vi "observacao.vi"() -> ()   [LabVIEW 2018, in "Shared_160.lvlib"] (continued)
                        n701 = call "Monta Comando.vi"("Comando"="ABRIR", "Dispositivo"="TRAPEIRA" ("Comando"), "Controlador"=w615) -> ()  [unwired: 2 in, 5 out]
                      }
                      frame True {
                        # "CLP Busy"
                        n702 = local read "TimeoutCUP"() -> (w618:u32)
                        n703 = call "TickTimeout.vi"("msInicial"=w618, "msTimeout"=u32 5000) -> ("Timeout"=w617:bool)  [unwired: 2 out]
                        n704 = case shown="True" w617 {
                          tunnel: [6 3] -> w616
                          frame False {
                          }
                          frame True {
                          }
                        }
                      }
                    }
                  }
                }
              }
              frame 7 {
                w622 = u16 15 items=["Alarme", "Atencao", "Erro", "Ocupado", "Plataforma", "LCB", "Trapeira", "Paravento", "DomoRap", "DomoCW", "DomoCCW", "TBD", "Em movimento", "TrapRUN", "TrapFCH", "TrapABT"] ("NomeStatus")
                # "Aqui também caberia um Timeout?"
                # "Aguarda abertura Trapeira"
                n705 = call "Bit Status CUP.vi"("NomeStatus"=w622) -> ("StatBit"=w623:bool)
                n706 = case shown="True" w623 {
                  tunnel: [7 0] -> w624
                  frame False {
                    # "Ainda movendo...\nAGUARDAR"
                  }
                  frame True {
                    # "Trapeira aberta.\nFIM"
                    n707 = call "TickTimeout.vi"() -> ("msTick"=w626:u32)  [unwired: 2 in, 2 out]
                    n708 = local write "Dome on Target"(TRUE ("Dome on Target")) -> ()
                    n709 = local write "TimeoutCUP"(w626) -> ()
                    n710 = global write "Global_Telescopio.vi" "T cup"(w626) -> ()
                  }
                }
              }
            }
            n711 = Equal To 0?(x=w493) -> (x = 0?=w492:bool)
            n712 = And(x=w492, y=w477) -> (x .and. y?=w488:bool)
            n713 = case shown="True" w488 {
              tunnel: w477 -> [w506 _]
              tunnel: [w505 "POINT" ("Boolean Text.Text")] -> w476
              frame False {
                n714 = case shown="True" w506 {
                  tunnel: ["POINT" ("Boolean Text.Text") "STOP" ("Boolean Text.Text")] -> w505
                  frame False {
                  }
                  frame True {
                  }
                }
              }
              frame True {
                w509 = TRUE
                # "MUDANÇA:\n22/6/2011 \nHab. Guider"
                n715 = local read "ChkDomeEnable"() -> (w510:bool)
                n716 = global write "Global_Telescopio.vi" "Botão GO = STOP"(FALSE) -> ()
                n717 = local write "LED GUIDER"(w509) -> ()
                n718 = local write "GUIDER"(w509) -> ()
                n719 = local write "DOME"(w510) -> ()
              }
            }
            n720 = Tick Count (ms)() -> (millisecond timer value=w469:u32)
            n721 = Subtract(x=w469, y=w475) -> (x-y=w468:u32)
            n722 = Less?(x=w468, y=w470) -> (x < y?=w471:bool)
            n723 = case shown="True" w471 {
              tunnel: w470 -> [_ w504]
              frame False {
              }
              frame True {
                n724 = Wait Until Next ms Multiple(millisecond multiple=w504) -> ()  [unwired: 1 out]
              }
            }
            n725 = control-ref of="BtTargetPoint"() -> (w503:refnum<vi>)
            n726 = call "PROTECAO.vi"("Estado In"=w481) -> ("Estado Out"=w480:i32)  [unwired: 2 in]
            n727 = property class="Bool"(reference=w503, "Boolean Text.Text"=w476) -> ()  [unwired: 1 in, 2 out]
            n728 = local write "statCUP"(w480) -> ()
            "statCUP 2" <- "statCUP"
            "Erro Lim" <- 15 ("y")
            "Erro PROTEC" <- 10 ("y")
          }
          frame #4 {
            # "CHECA FINAL DO APONTAMENTO"
            # "ascensão reta = tempo sideral - ângulo horário (2)"
            n729 = local read "LedPointing"() -> (w937:bool)
            n730 = case shown="True" w937 {
              frame False {
                n731 = property on="DOME" class="Bool (strict)"("Disabled"=u8 0) -> ()  [unwired: 2 in, 2 out]
              }
              frame True {
                n732 = local read "statCUP"() -> (w942:i32)
                n733 = local read "statAH"() -> (w941:i32)
                n734 = local read "statDEC"() -> (w943:i32)
                n735 = Compound Arithmetic op=ADD(w942, w941, w943) -> (w944:i32)
                n736 = Greater Than 0?(x=w944) -> (x > 0?=w940:bool)
                n737 = case shown="False" w940 {
                  selector: w940 -> [w945 _]
                  frame False {
                    w948 = TRUE
                    n738 = local read "ChkPointPrecessed"() -> (w946:bool)
                    n739 = local read "StrPointObjName"() -> (w951:string)
                    n740 = local read "StrPointObjRA"() -> (w950:string)
                    n741 = local read "StrPointObjDEC"() -> (w949:string)
                    n742 = local write "LedPointing"(w945) -> ()
                    n743 = property on="LedPointing" class="Bool (strict)"("Visible"=w945) -> ()  [unwired: 2 in, 2 out]
                    n744 = case shown="True" w946 {
                      tunnel: ["2000.000000000" ("Saída") w953] -> w947
                      frame False {
                        # "20240805"
                      }
                      frame True {
                        # "20240805"
                        n745 = call "Calcula epoch.vi"() -> ("epoch"=w956:dbl)  [unwired: 2 in]
                        n746 = Number To Fractional String(number=w956, precision (6)=i16 9) -> (F-format string=w954:string)  [unwired: 2 in]
                        n747 = call "Comma_to_Point.vi"("Lat_A"=w954) -> ("Saída"=w953:string)
                      }
                    }
                    n748 = global write "Global_Telescopio.vi" "NAME OBJETO"(w951) -> ()
                    n749 = global write "Global_Telescopio.vi" "DEC AQUIS"(w949) -> ()
                    n750 = global write "Global_Telescopio.vi" "RA AQUIS"(w950) -> ()
                    n751 = local write "Processa Centragem"(w948) -> ()
                    n752 = property on="LedPointWorkArea" class="Bool (strict)"("Visible"=w948) -> ()  [unwired: 2 in, 2 out]
                    n753 = global write "Global_Telescopio.vi" "EPOCH AQUIS"(w947) -> ()
                  }
                  frame True {
                  }
                }
              }
            }
            n754 = local read "VARIABLE \nTRACKING"() -> (w938:bool)
            n755 = case shown="True" w938 {
              frame False {
              }
              frame True {
                n756 = local write "DEC"("DECTARGET") -> ()
                n757 = local write "RA"("AHTARGET") -> ()
              }
            }
          }
          frame #5 {
            # "PROCESSO OBJETO CENTRADO"
            n758 = case shown="True" "Processa Centragem" {
              frame False {
              }
              frame True {
                w965 = u16 3 items=["Alarme", "Atencao", "Erro", "Ocupado", "Protecao", "Embreagem", "Tracking", "Var. Track", "Rápido", "Ligeiro", "Médio", "Lento", "Em movimento", ""] ("NomeStatus")
                w966 = u16 3 items=["Alarme", "Atencao", "Erro", "Ocupado", "Protecao", "Embreagem", "Tracking", "Var. Track", "Rápido", "Ligeiro", "Médio", "Lento", "Em movimento", ""] ("NomeStatus")
                # "Roda case interno quando \nos controladores AH e DEC\nestiverem desocupados."
                n759 = call "Bit Status AH.vi"("NomeStatus"=w966) -> ("StatBit"=w964:bool)
                n760 = call "Bit Status DEC.vi"("NomeStatus"=w965) -> ("StatBit"=w963:bool)
                n761 = Or(x=w964, y=w963) -> (x .or. y?=w960:bool)
                n762 = case shown="False" w960 {
                  selector: w960 -> [w985 _]
                  tunnel: "INDEXER" ("Comando") -> [w987 _]
                  tunnel: "ZERAR" ("Comando") -> [w986 _]
                  frame False {
                    w973 = u16 1 items=["ZERO", "AH", "DEC", "TUBO", "CUP"] ("Controlador")
                    w974 = u16 2 items=["ZERO", "AH", "DEC", "TUBO", "CUP"] ("Controlador")
                    w967 = 0.0 ("AcumAG DEC")
                    # "PROCESSOPRECESSÃO"
                    # "PROCESSO ZERA POS_MOTOR"
                    # "Precessão"
                    n763 = local read "PM_RA"() -> (w979:string)
                    n764 = local read "Temp amb"() -> (w982:string)
                    n765 = local read "hum local"() -> (w980:string)
                    n766 = local read "MeanDEC"() -> (w983:string)
                    n767 = local read "pressão atm"() -> (w981:string)
                    n768 = local read "MeanRA"() -> (w984:string)
                    n769 = local read "PM_DEC"() -> (w978:string)
                    n770 = call "Monta Comando.vi"("Comando"=w986, "Dispositivo"=w987, "Controlador"=w973) -> ()  [unwired: 2 in, 5 out]
                    n771 = call "Monta Comando.vi"("Comando"=w986, "Dispositivo"=w987, "Controlador"=w974) -> ()  [unwired: 2 in, 5 out]
                    n772 = call "PrecessFortran.vi"("Asc reta"=w984, "Var RA"=w979, "Declinação"=w983, "Temperatura (Kelvin)"=w982, "Pressao atmosferica (mB)"=w981, "Humidade relativa (0 a 1)"=w980, "Var DEC"=w978) -> ("Observed RA (radians)"=w977:dbl, "Observed Dec (radians)"=w976:dbl)  [unwired: 2 in, 5 out]
                    n773 = local write "Processa Centragem"(w985) -> ()
                    n774 = global write "Global_Telescopio.vi" "LatchPrecRA"(w977) -> ()
                    n775 = global write "Global_Telescopio.vi" "LatchPrecDEC"(w976) -> ()
                    n776 = global read "Global_Telescopio.vi" "Sideral Time"() -> (w970:dbl)
                    n777 = global read "Global_Telescopio.vi" "PosDEC"() -> (w972:dbl)
                    n778 = global read "Global_Telescopio.vi" "PosAH"() -> (w971:dbl)
                    n779 = Subtract(x=w970, y=w971) -> (x-y=w969:dbl)
                    n780 = local write "LatchDeslocDEC"(w972) -> ()
                    n781 = local write "LatchDeslocRA"(w969) -> ()
                    n782 = global write "Global_Telescopio.vi" "AcumPrecDEC"(w967) -> ()
                    n783 = global write "Global_Telescopio.vi" "LatchAG RA"(w967) -> ()
                    n784 = global write "Global_Telescopio.vi" "AcumAG DEC"(w967) -> ()
                    n785 = global write "Global_Telescopio.vi" "AcumPrecRA"(w967) -> ()
                    n786 = global write "Global_Telescopio.vi" "LatchAG DEC"(w967) -> ()
                    n787 = global write "Global_Telescopio.vi" "AcumAG RA"(w967) -> ()
                    n788 = global write "Global_Telescopio.vi" "ObjCentrado"(TRUE) -> ()
                    n789 = property on="Calagem" class="Bool"("Disabled"=u8 0) -> ()  [unwired: 2 in, 2 out]
                  }
                  frame True {
                  }
                }
              }
            }
          }
          frame #6 {
            w991 = u16 2 items=["Alarme", "Atencao", "Erro", "Ocupado", "TBD", "LCB", "Trapeira", "Paravento", "DomoRap", "DomoCW", "DomoCCW", "TBD", "Em movimento", "TBD"] ("NomeStatus")
            w992 = u16 3 items=["Alarme", "Atencao", "Erro", "Ocupado", "TBD", "LCB", "Trapeira", "Paravento", "DomoRap", "DomoCW", "DomoCCW", "TBD", "Em movimento", "TBD"] ("NomeStatus")
            w996 = u16 3 items=["Alarme", "Atencao", "Erro", "Ocupado", "Protecao", "Embreagem", "Tracking", "Var. Track", "Rápido", "Ligeiro", "Médio", "Lento", "Em movimento", ""] ("NomeStatus")
            w997 = u16 3 items=["Alarme", "Atencao", "Erro", "Ocupado", "Protecao", "Embreagem", "Tracking", "Var. Track", "Rápido", "Ligeiro", "Médio", "Lento", "Em movimento", ""] ("NomeStatus")
            w1005 = "ERROS" ("Comando")
            w1008 = u16 2 items=["Alarme", "Atencao", "Erro", "Ocupado", "Protecao", "Embreagem", "Tracking", "Var. Track", "Rápido", "Ligeiro", "Médio", "Lento", "Em movimento", ""] ("NomeStatus")
            w1009 = u16 2 items=["Alarme", "Atencao", "Erro", "Ocupado", "Protecao", "Embreagem", "Tracking", "Var. Track", "Rápido", "Ligeiro", "Médio", "Lento", "Em movimento", ""] ("NomeStatus")
            w1006 = "PROG" ("Comando")
            # "LOGTCS ERROS"
            n790 = call "Bit Status AH.vi"("NomeStatus"=w1009) -> ("StatBit"=w999:bool)
            n791 = call "Bit Status AH.vi"("NomeStatus"=w997) -> ("StatBit"=w995:bool)
            n792 = call "Bit Status DEC.vi"("NomeStatus"=w1008) -> ("StatBit"=w998:bool)
            n793 = call "Bit Status DEC.vi"("NomeStatus"=w996) -> ("StatBit"=w994:bool)
            n794 = call "Bit Status CUP.vi"("NomeStatus"=w991) -> ("StatBit"=w1007:bool)
            n795 = call "Bit Status CUP.vi"("NomeStatus"=w992) -> ("StatBit"=w1004:bool)
            n796 = Not(x=w1004) -> (.not. x?=w1003:bool)
            n797 = Not(x=w995) -> (.not. x?=w1001:bool)
            n798 = Not(x=w994) -> (.not. x?=w1002:bool)
            n799 = And(x=w1007, y=w1003) -> (x .and. y?=w990:bool)
            n800 = And(x=w999, y=w1001) -> (x .and. y?=w1000:bool)
            n801 = And(x=w998, y=w1002) -> (x .and. y?=w993:bool)
            n802 = And(x=FALSE, y=w990) -> (x .and. y?=w989:bool)
            n803 = case shown="True" w993 {
              selector: w993 -> [_ w1018]
              tunnel: w1006 -> [_ w1019]
              tunnel: w1005 -> [_ w1015]
              frame False {
              }
              frame True {
                w1016 = u16 2 items=["ZERO", "AH", "DEC", "TUBO", "CUP"] ("Controlador")
                n804 = call "Monta Comando.vi"("Comando"=w1015, "Dispositivo"=w1019, "Controlador"=w1016) -> ("Resposta"=w1017:string)  [unwired: 2 in, 4 out]
                n805 = call "Envia LOG.vi"("Error message"=w1017, "Controlador"=w1016, "Log de erro"=w1018) -> ()  [unwired: 5 in, 2 out]
              }
            }
            n806 = case shown="True" w989 {
              selector: w989 -> [_ w1013]
              tunnel: w1006 -> [_ w1014]
              tunnel: w1005 -> [_ w1010]
              frame False {
              }
              frame True {
                w1011 = u16 4 items=["ZERO", "AH", "DEC", "TUBO", "CUP"] ("Controlador")
                n807 = call "Monta Comando.vi"("Comando"=w1010, "Dispositivo"=w1014, "Controlador"=w1011) -> ("Resposta"=w1012:string)  [unwired: 2 in, 4 out]
                n808 = call "Envia LOG.vi"("Error message"=w1012, "Controlador"=w1011, "Log de erro"=w1013) -> ()  [unwired: 5 in, 2 out]
              }
            }
            n809 = case shown="True" w1000 {
              selector: w1000 -> [_ w1023]
              tunnel: w1006 -> [_ w1024]
              tunnel: w1005 -> [_ w1020]
              frame False {
              }
              frame True {
                w1021 = u16 1 items=["ZERO", "AH", "DEC", "TUBO", "CUP"] ("Controlador")
                n810 = call "Monta Comando.vi"("Comando"=w1020, "Dispositivo"=w1024, "Controlador"=w1021) -> ("Resposta"=w1022:string)  [unwired: 2 in, 4 out]
                n811 = call "Envia LOG.vi"("Error message"=w1022, "Controlador"=w1021, "Log de erro"=w1023) -> ()  [unwired: 5 in, 2 out]
              }
            }
          }
          frame #7 {
            # "MASSA DE AR"
            # "z'"
            # "z * (1 - 0,0012* (z* z -1) )"
            # "(z* z -1)"
            # "z"
            # "O Hour Angle é calculado com essa equação (AH = TS - RA), \nsendo TS o tempo sideral que você fica calculando o tempo todo e RA a \ncoordenada que vem do quadro TARGET da aba POINTING."
            # "Coslat"
            # "Sinlat"
            # "MASSA DE AR\n# define LAT -22,534444444444 / / Lat itude do telescópio\n# define SINLAT -0,383238771 / / Seno da Lat itude\n# define COSLAT 0,923649308 / / Cosseno da Lat itude\ndouble airmass (double ah, double delta) / / ângulos dos eixos AH e DEC em radianos\n{ double z;\nz = 1./ (SINLAT* sin(delta) + COSLAT* cos(delta) * cos(ah) ) ;\nz = z * (1 - 0,0012* (z* z -1) ) ;\nif (z > = 10) z = 9.999;\nif (z < 0) z = 0;\nreturn (z) ;\n}"
            n812 = global read "Global_Telescopio.vi" "AH_now"() -> (w1025:dbl)
            n813 = global read "Global_Telescopio.vi" "delta_now"() -> (w1026:dbl)
            n814 = Cosine(x=w1026) -> (cos(x)=w1046:dbl)
            n815 = Sine(x=w1026) -> (sin(x)=w1048:dbl)
            n816 = Cosine(x=w1025) -> (cos(x)=w1044:dbl)
            n817 = Multiply(x=0.923649308 ("Delta=DEC"), y=w1046) -> (x*y=w1045:dbl)
            n818 = Multiply(x=-0.383238771 ("Delta=DEC"), y=w1048) -> (x*y=w1043:dbl)
            n819 = Multiply(x=w1045, y=w1044) -> (x*y=w1042:dbl)
            n820 = Add(x=w1043, y=w1042) -> (x+y=w1041:dbl)
            n821 = Reciprocal(x=w1041) -> (1/x=w1033:dbl)
            n822 = Subtract(x=w1033, y=1.0) -> (x-y=w1039:dbl)
            n823 = Multiply(x=w1033, y=w1039) -> (x*y=w1038:dbl)
            n824 = Multiply(x=w1038, y=0.0012) -> (x*y=w1035:dbl)
            n825 = Subtract(x=1.0 ("y"), y=w1035) -> (x-y=w1034:dbl)
            n826 = Multiply(x=w1033, y=w1034) -> (x*y=w1030:dbl)
            n827 = Greater Or Equal?(x=w1030, y=10.0) -> (x >= y?=w1031:bool)
            n828 = case shown="True" w1031 {
              tunnel: [w1052 9.999999 ("y")] -> w1028
              tunnel: w1030 -> [w1052 _]
              frame False {
              }
              frame True {
              }
            }
            n829 = Less Than 0?(x=w1028) -> (x < 0?=w1029:bool)
            n830 = case shown="True" w1029 {
              tunnel: [w1050 0.0 ("y")] -> w1027
              tunnel: w1028 -> [w1050 _]
              frame False {
              }
              frame True {
              }
            }
            "Air Mass" <- w1027
            n831 = global write "Global_Telescopio.vi" "Air Mass"(w1027) -> ()
          }
          frame #8 {
          }
          frame #9 {
            # "20250707"
            # "ZeroMQ"
            # "ZeroMQ"
            # "CONDIÇÕES ATMOSFÉRICAS"
            # "A cada n Segundos\nEssa rotina gera 1\npulso!"
            # "Seg"
            # "Janela Das Condições Atmosféricas"
            n832 = property on="Weather data received" class="Bool (strict)"() -> ("Blinking"=w1056:bool)  [unwired: 2 in, 2 out]
            n833 = local write "Weather data received"(w1056) -> ()
            n834 = call "Get weather data.vi"() -> ("Wather160 data"=w1057:string[])  [unwired: 9 in]
            n835 = call "timepulse.vi"("de quantos segundos"=i16 10) -> ("PULSO"=w1061:bool)  [unwired: 2 in]
            n836 = call "Pulso_se_Mudou.vi"("Entrada"="Int/Ext") -> ("Saída"=w1059:bool)
            n837 = And(x="Int/Ext", y=w1061) -> (x .and. y?=w1058:bool)
            n838 = case shown="True" w1058 {
              tunnel: [TRUE TRUE ("Int/Ext")] -> w1055
              tunnel: w1059 -> [w1071 _]
              tunnel: w1057 -> [w1070 w1095]
              frame False {
                # "A chave Int/Ext mudou\npara pushbutton e é tratada apenas dentro deste case \"False\" nos períodos inativos de \"time pulse\" ligado ao terminal ? do case.\n\nOs valores internos (dew point, temperatura, umidade ) somente são mostrados enquanto a chave ficar pressionada pelo mouse.\n\nIsto garante o uso dos valores externos desssas grandezas no cálculo da precessão."
                n839 = case shown="True" w1071 {
                  tunnel: w1070 -> [_ w1072]
                  frame False {
                  }
                  frame True {
                    # "ZeroMQ"
                    # "Display"
                    # "ESTE CASO SOMENTE É EXECUTADO QUANDO A CHAVE INT/EXT MUDA DE ESTADO"
                    n840 = local read "Int/Ext"() -> (w1076:bool)
                    n841 = case shown="True" w1076 {
                      tunnel: [28 ("index") 5 ("index")] -> w1074
                      tunnel: [29 ("index") 6 ("index")] -> w1075
                      tunnel: [27 ("index") 2 ("index")] -> w1073
                      frame False {
                        # "Interno"
                      }
                      frame True {
                        # "Externo"
                      }
                    }
                    n842 = Index Array(array=w1072, index #1=w1073, index #2=w1074, index #3=w1075) -> (element #1=w1079:string, element #2=w1078:string, element #3=w1077:string)
                    n843 = call "point_to_comma.vi"("Lat_A"=w1079) -> ("Saída"=w1081:string)
                    n844 = call "point_to_comma.vi"("Lat_A"=w1078) -> ("Saída"=w1082:string)
                    n845 = call "point_to_comma.vi"("Lat_A"=w1077) -> ("Saída"=w1085:string)
                    n846 = Fract/Exp String To Number(string=w1081, default (0 dbl)=1.0 ("default (0 DBL)")) -> (number=w1086:dbl)  [unwired: 2 in, 1 out]
                    n847 = Fract/Exp String To Number(string=w1082, default (0 dbl)=1.0 ("default (0 DBL)")) -> (number=w1087:dbl)  [unwired: 2 in, 1 out]
                    n848 = Fract/Exp String To Number(string=w1085, default (0 dbl)=1.0 ("default (0 DBL)")) -> (number=w1088:dbl)  [unwired: 2 in, 1 out]
                    n849 = local write "Temperature"(w1086) -> ()
                    n850 = local write "Humidity"(w1087) -> ()
                    n851 = local write "Dew Point"(w1088) -> ()
                  }
                }
              }
              frame True {
                n852 = stacked-sequence {
                  tunnel: w1095 -> [_ w1115 _ _]
                  frame #0 {
                    # "O botão INT/ EXT (cf. figura 3) seleciona se os most radores TEMPERATURE, HUMIDITY\ne DEW POINT são atualizados com os valores internos ou externos desse regist ro.\nA barra gráfica CLOUSURE LIMITS deve ser deslocada em função da proximidade\n(dada por um valor percentural de zero a 100%) dos valores lidos do arquivo de dados\natmosféricos com os valores- limite das grandezas listadas nesse quadro. Para\nPRESSURE e WIND SPEED, considerar os valores- limite desse quadro como o final de\numa escala de 0 a 100%, cujo valor inicial (0%) corresponde ao valor zero dessas\ngrandezas. Para as grandezas DEWPOINT, interna e externa, considerar os valores\nlimites listados no quadro como final da escala (100%) e cada décimo de ºC acima\ndos valores- limite como 1% da escala."
                    # "A simulação da janela ENVIRONMENT STATUS será feita com os dados de um arquivo\ngerado pela estação meteorológica contendo os regist ros de 24 horas de monitoria,\nsendo cada regist ro efetuado em intervalos de 10 minutos. A simulação deve procurar\nnesse arquivo (anexo, LNA-TCSPD-MP-00012-01-100.txt ) o regist ro correspondente à\nhora local do PC, ler esse regist ro e ret irar as informações de cada most rador para\natualizar essa janela."
                  }
                  frame #1 {
                    w1139 = "\t"
                    # "ZeroMQ"
                    # "O Fortran usa valores\nde umidade entre 0 e 1."
                    # "MUDANÇA 08/04/2011:\nCriada a variável AtmosferaStr para guardar dados\nmeteorológicos para Erros de Apontamento"
                    # "Celsius -->Kelvin\nO Fortran usa Kelvin"
                    # "bar"
                    n853 = global read "Global_Telescopio.vi" "weather160 PUB time"() -> (→"Weather rec. time":timestamp)
                    n854 = case shown="True" TRUE {
                      tunnel: [27 ("index") 2 ("index")] -> w1133
                      tunnel: [28 ("index") 5 ("index")] -> w1132
                      tunnel: [29 ("index") 6 ("index")] -> w1131
                      frame False {
                        # "Interno"
                      }
                      frame True {
                        # "Externo"
                      }
                    }
                    n855 = global read "Global_Telescopio.vi" "Default Met"() -> (w1108:bool)
                    n856 = Index Array(array=w1115, index #1=w1133, index #2=w1132, index #3=w1131, index #4=7 ("index"), index #5=8 ("index"), index #6=12 ("index"), index #7=16 ("index"), index #8=2 ("index"), index #9=5 ("index"), index #10=27 ("index"), index #11=28 ("index"), index #12=35 ("index")) -> (element #1=w1164:string, element #2=w1176:string, element #3=w1173:string, element #4=w1169:string, element #5=w1140:string, element #6=w1168:string, element #7=w1113:string, element #8=w1112:string, element #9=w1111:string, element #10=w1150:string, element #11=w1149:string, element #12=w1134:string)
                    "Wind Dir" <- w1140
                    n857 = property on="Default" class="Str"("Visible"=w1108) -> ()  [unwired: 2 in, 2 out]
                    n858 = call "Weather data mabager.vi"("umidade in"=w1111, "temperatura in"=w1112, "pressao in"=w1113, "Default Met"=w1108) -> ("umidade out"=w1109:string, "temperatura out"=w1110:string, "pressao out"=w1114:string, "led on"=→"Weather data received":bool, "wather160 led state"=w1104:cluster{u32, u32}[], "blink"=w1105:bool)  [unwired: 2 out]
                    n859 = property on="Weather data received" class="Bool (strict)"("Colors [4]"=w1104) -> ()  [unwired: 2 in, 2 out]
                    n860 = property on="Weather data received" class="Bool (strict)"("Blinking"=w1105) -> ()  [unwired: 2 in, 2 out]
                    n861 = Decimal String To Number(string=w1134) -> (number=→"LEAF":i32)  [unwired: 2 in, 1 out]
                    n862 = call "point_to_comma.vi"("Lat_A"=w1164) -> ("Saída"=w1161:string)
                    n863 = call "point_to_comma.vi"("Lat_A"=w1176) -> ("Saída"=w1162:string)
                    n864 = call "point_to_comma.vi"("Lat_A"=w1173) -> ("Saída"=w1143:string)
                    n865 = call "point_to_comma.vi"("Lat_A"=w1169) -> ("Saída"=w1141:string)
                    n866 = call "point_to_comma.vi"("Lat_A"=w1168) -> ("Saída"=w1142:string)
                    n867 = call "point_to_comma.vi"("Lat_A"=w1114) -> ("Saída"=w1146:string)
                    "pressão atm" <- w1146
                    n868 = call "point_to_comma.vi"("Lat_A"=w1113) -> ("Saída"=w1117:string)
                    n869 = call "point_to_comma.vi"("Lat_A"=w1110) -> ("Saída"=w1148:string)
                    n870 = call "point_to_comma.vi"("Lat_A"=w1109) -> ("Saída"=w1147:string)
                    n871 = call "point_to_comma.vi"("Lat_A"=w1150) -> ("Saída"=w1145:string)
                    n872 = call "point_to_comma.vi"("Lat_A"=w1149) -> ("Saída"=w1144:string)
                    n873 = Concatenate Strings(w1148, w1139, w1147, w1139, w1146, w1139, w1145, w1139, w1144, w1139, w1143, w1139, w1141, w1139, w1140, w1139) -> (→"AtmosferaStr":string)
                    n874 = Fract/Exp String To Number(string=w1117, default (0 dbl)=1.0 ("default (0 DBL)")) -> (number=→"Pressure":dbl)  [unwired: 2 in, 1 out]
                    n875 = Fract/Exp String To Number(string=w1161, default (0 dbl)=1.0 ("default (0 DBL)")) -> (number=→"Temperature":dbl)  [unwired: 2 in, 1 out]
                    n876 = Fract/Exp String To Number(string=w1162, default (0 dbl)=1.0 ("default (0 DBL)")) -> (number=→"Humidity":dbl)  [unwired: 2 in, 1 out]
                    n877 = Fract/Exp String To Number(string=w1143, default (0 dbl)=1.0 ("default (0 DBL)")) -> (number=→"Dew Point":dbl)  [unwired: 2 in, 1 out]
                    n878 = Fract/Exp String To Number(string=w1141, default (0 dbl)=1.0 ("default (0 DBL)")) -> (number=→"Wind Speed":dbl)  [unwired: 2 in, 1 out]
                    n879 = Fract/Exp String To Number(string=w1142, default (0 dbl)=1.0 ("default (0 DBL)")) -> (number=→"Wind Chill":dbl)  [unwired: 2 in, 1 out]
                    n880 = Fract/Exp String To Number(string=w1146, default (0 dbl)=1.0 ("default (0 DBL)")) -> (number=w1135:dbl)  [unwired: 2 in, 1 out]
                    n881 = Fract/Exp String To Number(string=w1148, default (0 dbl)=1.0 ("default (0 DBL)")) -> (number=w1120:dbl)  [unwired: 2 in, 1 out]
                    n882 = Fract/Exp String To Number(string=w1147, default (0 dbl)=1.0 ("default (0 DBL)")) -> (number=w1119:dbl)  [unwired: 2 in, 1 out]
                    n883 = Add(x=w1120, y=273.5 ("default (0 DBL)")) -> (x+y=w1159:dbl)
                    n884 = Divide(x=w1119, y=100.0 ("default (0 DBL)")) -> (x/y=w1153:dbl)
                    n885 = global write "Global_Telescopio.vi" "BAR"(w1135) -> ()
                    n886 = global write "Global_Telescopio.vi" "HUM"(w1119) -> ()
                    n887 = global write "Global_Telescopio.vi" "TEMP"(w1120) -> ()
                    n888 = Number To Fractional String(number=w1159, precision (6)=i16 1) -> (F-format string=→"Temp amb":string)  [unwired: 2 in]
                    n889 = Number To Fractional String(number=w1153, precision (6)=i16 2) -> (F-format string=→"hum local":string)  [unwired: 2 in]
                    n890 = call "Alarme_Atmosferico.vi"("Internal Dew Point"="Internal Dew Point", "Dew Point"="Dew Point 2", "Humidity"="Humidity 2", "Wind Speed"="Wind Speed 2", "LEAF"="LEAF 2") -> ("PUB alarme atmosferico"=w1097:string)  [unwired: 6 in]
                    n891 = global write "Global_Telescopio.vi" "PUB AtmAlarme"(w1097) -> ()
                  }
                  frame #2 {
                    # "Em relação as suas perguntas:\n- Temperaturas (Temperature, Dew Point e Wind Chill): mínimo/máximo: -20 a +50 graus\n- Humidity:  0 a 100%\n- Pressão atmosférica: de 300 a 1200 mBar\n- Velocidade do vento: 0 a 300 Km/h\n\nNotar que a chave INT/EXT na parte superior do quadro \nesquerdo seleciona se são mostrados os valores internos ou externos de Temperatura, Umidade e Dew Point."
                    # "Pressure Max"
                    # "Wind chill Point Max"
                    # "Temp Point Max"
                    # "Dew Point Max"
                    # "Humidity Max"
                    # "Speed Max"
                    # "Steady Wind           >  70 Km/h\nRelative Humidity    >  97 %\nInternal Dewpoint  <  0.5  C\nExternal Dewpoint <  1.0  C"
                    n892 = Divide(x=100.0, y=300.0 ("x")) -> (x/y=w1214:dbl)
                    n893 = Divide(x=100.0, y=100.0 ("x")) -> (x/y=w1208:dbl)
                    n894 = Divide(x=100.0, y=50.0 ("x")) -> (x/y=w1206:dbl)
                    n895 = Divide(x=100.0, y=50.0 ("x")) -> (x/y=w1200:dbl)
                    n896 = Divide(x=100.0, y=50.0 ("x")) -> (x/y=w1199:dbl)
                    n897 = Divide(x=100.0, y=1200.0 ("x")) -> (x/y=w1194:dbl)
                    n898 = local read "Temperature"() -> (w1191:dbl)
                    n899 = local read "Wind Speed"() -> (w1213:dbl)
                    n900 = local read "Wind Chill"() -> (w1192:dbl)
                    n901 = local read "Dew Point"() -> (w1203:dbl)
                    n902 = local read "Humidity"() -> (w1207:dbl)
                    n903 = local read "Pressure"() -> (w1193:dbl)
                    n904 = Multiply(x=w1213, y=w1214) -> (x*y=w1190:dbl)
                    n905 = Multiply(x=w1207, y=w1208) -> (x*y=w1189:dbl)
                    n906 = Multiply(x=w1203, y=w1206) -> (x*y=w1188:dbl)
                    n907 = Multiply(x=w1191, y=w1200) -> (x*y=w1187:dbl)
                    n908 = Multiply(x=w1192, y=w1199) -> (x*y=w1186:dbl)
                    n909 = Multiply(x=w1193, y=w1194) -> (x*y=w1185:dbl)
                    n910 = Build Array(w1190, w1189, w1188, w1187, w1186, w1185) -> (w1184:dbl[])
                    n911 = Array Max & Min(array=w1184) -> (max value=w1183:dbl)  [unwired: 3 out]
                    n912 = local write "SlideEnviromental"(w1183) -> ()
                  }
                  frame #3 {
                    # "Determinadas as proximidades de cada grandeza em valores percentuais, selecionar o\nvalor da mais elevada para ser most rado na barra gráfica. A cor dessa barra gráfica\ndeve mudar em função do valor most rado. Enquanto est iver abaixo de 90%, ela deve\nser verde, ent re 90 e 95% amarela e acima de 95% vermelha. O led ao lado desse\nbarra deve ficar ligado e ter a mesma cor da barra gráfica, mas quando esta\nult rapassar 90%, ou seja quando for amarela ou vermelha, o led deve piscar."
                    n913 = local read "SlideEnviromental"() -> (w1215:dbl)
                    n914 = In Range and Coerce(upper limit=95.0 ("lower limit"), x=w1215, lower limit=90.0 ("upper limit")) -> (In Range?=w1220:bool)  [unwired: 1 out]
                    n915 = Less?(x=w1215, y=90.0) -> (x < y?=w1222:bool)
                    n916 = Greater?(x=w1215, y=95.0 ("lower limit")) -> (0:w1219:bool)
                    n917 = case shown="True" w1220 {
                      frame False {
                      }
                      frame True {
                        n918 = stacked-sequence {
                          frame #0 {
                            n919 = property on="SlideEnviromental" class="Slide (strict)"("Fill Color"=u32 16772882) -> ()  [unwired: 2 in, 2 out]
                            n920 = local write "Boolean 11"(TRUE ("Boolean 11")) -> ()
                            n921 = property on="Boolean 11" class="Bool (strict)"("Blinking"=FALSE) -> ()  [unwired: 2 in, 2 out]
                          }
                          frame #1 {
                            # "Cor do Led"
                            # "lig"
                            # "des"
                            n922 = Bundle(u32 7171459, u32 46096) -> (w1242:cluster{u32, u32})  [unwired: 1 in]
                            n923 = Bundle(u32 16772882, u32 46096) -> (w1241:cluster{u32, u32})  [unwired: 1 in]
                            n924 = Build Array(w1242, w1241) -> (w1240:cluster{u32, u32}[])
                            n925 = property on="Boolean 11" class="Bool (strict)"("Colors [4]"=w1240) -> ()  [unwired: 2 in, 2 out]
                          }
                        }
                      }
                    }
                    n926 = case shown="True" w1222 {
                      frame False {
                      }
                      frame True {
                        n927 = stacked-sequence {
                          frame #0 {
                            n928 = property on="SlideEnviromental" class="Slide (strict)"("Fill Color"=u32 6618880) -> ()  [unwired: 2 in, 2 out]
                            n929 = local write "Boolean 11"(TRUE ("Boolean 11")) -> ()
                            n930 = property on="Boolean 11" class="Bool (strict)"("Blinking"=FALSE) -> ()  [unwired: 2 in, 2 out]
                          }
                          frame #1 {
                            # "Cor do Led"
                            # "lig"
                            # "des"
                            n931 = Bundle(u32 7171459, u32 46096) -> (w1246:cluster{u32, u32})  [unwired: 1 in]
                            n932 = Bundle(u32 6618880, u32 46096) -> (w1247:cluster{u32, u32})  [unwired: 1 in]
                            n933 = Build Array(w1246, w1247) -> (w1248:cluster{u32, u32}[])
                            n934 = property on="Boolean 11" class="Bool (strict)"("Colors [4]"=w1248) -> ()  [unwired: 2 in, 2 out]
                          }
                        }
                      }
                    }
                    n935 = case shown="True" w1219 {
                      frame False {
                      }
                      frame True {
                        n936 = stacked-sequence {
                          frame #0 {
                            n937 = local write "Boolean 11"(TRUE ("Boolean 11")) -> ()
                            n938 = property on="SlideEnviromental" class="Slide (strict)"("Fill Color"=u32 16715776) -> ()  [unwired: 2 in, 2 out]
                            n939 = property on="Boolean 11" class="Bool (strict)"("Blinking"=TRUE) -> ()  [unwired: 2 in, 2 out]
                          }
                          frame #1 {
                            # "Cor do Led"
                            # "lig"
                            # "des"
                            n940 = Bundle(u32 7171459, u32 46096) -> (w1226:cluster{u32, u32})  [unwired: 1 in]
                            n941 = Bundle(u32 16715776, u32 46096) -> (w1227:cluster{u32, u32})  [unwired: 1 in]
                            n942 = Build Array(w1226, w1227) -> (w1228:cluster{u32, u32}[])
                            n943 = property on="Boolean 11" class="Bool (strict)"("Colors [4]"=w1228) -> ()  [unwired: 2 in, 2 out]
                          }
                        }
                      }
                    }
                  }
                }
              }
            }
            n944 = global read "Global_Telescopio.vi" "BtShutCloseSimul"() -> (w1054:bool)
            n945 = case shown="True" w1054 {
              frame False {
              }
              frame True {
                # "Escreve no LOG o estado do shutter"
                n946 = global write "Global_Telescopio.vi" "BtShutCloseSimul"(FALSE) -> ()
                n947 = call "Log_Shutter.vi"("command"=" ", "domeState"="CLOSED " ("command"), "pathLogDomeFile"="C:\\TCS\\LOG\\SHUTTER\\SHUTTER.TXT" ("pathLogFocoString")) -> ()  [unwired: 6 in]
              }
            }
            n948 = flat-sequence {
              tunnel: w1055 -> [_]
              frame #0 {
                n949 = local read "LEAF"() -> (w1068:i32)
                n950 = call "Testa_Leaf.vi"("enable"=TRUE, "LEAF"=w1068) -> ()  [unwired: 10 in]
              }
            }
          }
          frame #10 {
            w1276 = u16 3 items=["Alarme", "Atencao", "Erro", "Ocupado", "Protecao", "Embreagem", "Tracking", "Var. Track", "Rápido", "Ligeiro", "Médio", "Lento", "Em movimento", ""] ("NomeStatus")
            w1277 = u16 3 items=["Alarme", "Atencao", "Erro", "Ocupado", "Protecao", "Embreagem", "Tracking", "Var. Track", "Rápido", "Ligeiro", "Médio", "Lento", "Em movimento", ""] ("NomeStatus")
            # "20250728"
            # "PROCESSO AUTO GUIDER E NON-SIDERAL TRACKING"
            n951 = local read "ExternalTracking"() -> (w1259:bool)
            n952 = local read "VARIABLE \nTRACKING"() -> (w1254:bool)
            "LED VAR TRACKING" <- w1254
            n953 = global read "Global_Telescopio.vi" "ExtDEC correction"() -> (w1263:bool)
            n954 = global read "Global_Telescopio.vi" "ExtRA correction"() -> (w1262:bool)
            n955 = local read "MOUNT"() -> (w1269:bool)
            n956 = global read "Global_Telescopio.vi" "Correção Guider"() -> (w1273:bool)
            n957 = local read "LedPointing"() -> (w1275:bool)
            n958 = local read "MOVING"() -> (w1274:bool)
            n959 = call "Bit Status AH.vi"("NomeStatus"=w1277) -> ("StatBit"=w1266:bool)
            n960 = call "Bit Status DEC.vi"("NomeStatus"=w1276) -> ("StatBit"=w1265:bool)
            n961 = Not Or(1:w1265, 2:w1266) -> (0:w1270:bool)
            n962 = Not(x=w1274) -> (.not. x?=w1267:bool)
            n963 = Not(x=w1275) -> (.not. x?=w1268:bool)
            n964 = And(x=w1259, y=w1254) -> (x .and. y?=w1253:bool)
            "externalNST" <- w1253
            n965 = Or(x=w1263, y=w1262) -> (x .or. y?=w1264:bool)
            n966 = Not(x=w1259) -> (.not. x?=w1271:bool)
            n967 = global write "Global_Telescopio.vi" "PUB activeNST"(w1253) -> ()
            n968 = Compound Arithmetic op=AND(w1273, w1268, w1267, "GUIDER", w1269, w1270, w1271) -> (w1261:bool)
            n969 = Compound Arithmetic op=AND(w1269, w1268, w1267, w1259, w1254, w1264) -> (w1260:bool)
            n970 = case shown="True" w1261 {
              tunnel: w1260 -> [w1284 _]
              tunnel: w1266 -> [w1283 _]
              tunnel: w1265 -> [w1282 _]
              tunnel: w1263 -> [w1281 _]
              tunnel: w1262 -> [w1280 _]
              frame False {
                # "Reseta Flag da comunicação do Guider"
                # "CKECK FOR NON-SIDERAL TRACKING CORRECTIONS"
                n971 = case shown="True" w1284 {
                  tunnel: w1283 -> [_ w1291]
                  tunnel: w1282 -> [_ w1290]
                  tunnel: w1281 -> [_ w1289]
                  tunnel: w1280 -> [_ w1288]
                  frame False {
                    # "AO CONTRÁRIO DA CORREÇÃO GUIDER, O FLAG EXTERNAL CORRECTION NÃO DEVE SER APAGADO\nPARA SE TENTAR EXECUTAR A CORREÇÃO MAIS TARDE,, PARA NÃO PERDER O DESLOCAMENTO."
                    # "EXTERNAL NON-SIDERAL TRACKING DISABLED OR TELESCOPE NOT READY"
                  }
                  frame True {
                    # "EXTERNAL NON-SIDERAL TRACKING"
                    n972 = Not(x=w1291) -> (.not. x?=w1287:bool)
                    n973 = Not(x=w1290) -> (.not. x?=w1286:bool)
                    n974 = stacked-sequence {
                      tunnel: w1287 -> [w1294 _]
                      tunnel: w1286 -> [_ w1308]
                      tunnel: w1289 -> [_ w1309]
                      tunnel: w1288 -> [w1293 _]
                      frame #0 {
                        n975 = And(x=w1294, y=w1293) -> (x .and. y?=w1292:bool)
                        n976 = case shown="True" w1292 {
                          frame False {
                          }
                          frame True {
                            w1303 = u16 1 items=["ZERO", "AH", "DEC", "TUBO", "CUP"] ("Controlador")
                            # "MOVE TELESCÓPIO"
                            n977 = global read "Global_Telescopio.vi" "ExtRA_shift"() -> (w1299:string)
                            n978 = property on="Calagem" class="Bool"("Disabled"=u8 2) -> ()  [unwired: 2 in, 2 out]
                            n979 = call "Monta Comando.vi"("Set Point"=w1299, "Comando"="SHIFT", "Dispositivo"="EIXO" ("Comando"), "Controlador"=w1303) -> ("Erro Resp"=w1296:bool)  [unwired: 1 in, 4 out]
                            n980 = call "point_to_comma.vi"("Lat_A"=w1299) -> ("Saída"=w1298:string)
                            n981 = local read "Offset RA"() -> (w1301:dbl)
                            n982 = Fract/Exp String To Number(string=w1298) -> (number=w1297:dbl)  [unwired: 3 in, 1 out]
                            n983 = Add(x=w1297, y=w1301) -> (x+y=w1295:dbl)
                            n984 = case shown="False" w1296 {
                              selector: w1296 -> [w1305 _]
                              tunnel: w1295 -> [w1306 _]
                              frame False {
                                # "RESPOSTA ACK"
                                n985 = global write "Global_Telescopio.vi" "ExtRA correction"(w1305) -> ()
                                n986 = local write "Offset RA"(w1306) -> ()
                              }
                              frame True {
                                # "NAK"
                              }
                            }
                          }
                        }
                      }
                      frame #1 {
                        n987 = And(x=w1308, y=w1309) -> (x .and. y?=w1307:bool)
                        n988 = case shown="True" w1307 {
                          frame False {
                          }
                          frame True {
                            w1318 = u16 2 items=["ZERO", "AH", "DEC", "TUBO", "CUP"] ("Controlador")
                            # "MOVE TELESCÓPIO"
                            n989 = global read "Global_Telescopio.vi" "ExtDEC_shift"() -> (w1313:string)
                            n990 = property on="Calagem" class="Bool"("Disabled"=u8 2) -> ()  [unwired: 2 in, 2 out]
                            n991 = local read "Offset DEC"() -> (w1316:dbl)
                            n992 = call "Monta Comando.vi"("Set Point"=w1313, "Comando"="SHIFT", "Dispositivo"="EIXO" ("Comando"), "Controlador"=w1318) -> ("Erro Resp"=w1311:bool)  [unwired: 1 in, 4 out]
                            n993 = call "point_to_comma.vi"("Lat_A"=w1313) -> ("Saída"=w1314:string)
                            n994 = Fract/Exp String To Number(string=w1314) -> (number=w1312:dbl)  [unwired: 3 in, 1 out]
                            n995 = Add(x=w1312, y=w1316) -> (x+y=w1310:dbl)
                            n996 = case shown="False" w1311 {
                              selector: w1311 -> [w1320 _]
                              tunnel: w1310 -> [w1321 _]
                              frame False {
                                # "RESPOSTA ACK"
                                n997 = global write "Global_Telescopio.vi" "ExtDEC correction"(w1320) -> ()
                                n998 = local write "Offset DEC"(w1321) -> ()
                              }
                              frame True {
                                # "NAK"
                              }
                            }
                          }
                        }
                      }
                    }
                  }
                }
                n999 = global write "Global_Telescopio.vi" "Correção Guider"(FALSE ("Correção Guider")) -> ()
              }
              frame True {
                # "MUDANÇA:\n(25/08/2010)"
                # "É necessário testar se as\nstrings são igual a espaço\nem virtude de um BUG,\nno Soft do Auto guider!"
                # "TRADITIONAL GUIDING USING AUTOGUIDER"
                n1000 = global read "Global_Telescopio.vi" "guide_dir_ns"() -> (w1327:string)
                n1001 = global read "Global_Telescopio.vi" "guide_dir_we"() -> (w1328:string)
                n1002 = case shown="\"W\"" w1328 {
                  tunnel: [0.0 ("PreciseOffsetDEC 2") 1.0 ("PreciseOffsetDEC 2") -1.0 ("PreciseOffsetDEC 2")] -> w1325
                  frame " ", Default {
                  }
                  frame "W" {
                  }
                  frame "E" {
                  }
                }
                n1003 = case shown="\"N\"" w1327 {
                  tunnel: [0.0 ("PreciseOffsetDEC 2") 1.0 ("PreciseOffsetDEC 2") -1.0 ("PreciseOffsetDEC 2")] -> w1324
                  frame " ", Default {
                  }
                  frame "N" {
                  }
                  frame "S" {
                  }
                }
                n1004 = Equal To 0?(x=w1324) -> (x = 0?=w1323:bool)
                n1005 = Equal To 0?(x=w1325) -> (x = 0?=w1322:bool)
                n1006 = And(x=w1322, y=w1323) -> (x .and. y?=w1326:bool)
                n1007 = case shown="True" w1326 {
                  tunnel: w1325 -> [w1333 _]
                  tunnel: w1324 -> [w1332 _]
                  frame False {
                    # "Comandos do Auto guider contendo direção"
                    n1008 = global read "Global_Telescopio.vi" "esc_placa"() -> (w1331:string)
                    n1009 = Fract/Exp String To Number(use system decimal point (T)=FALSE, string=w1331) -> (number=w1330:dbl)  [unwired: 2 in, 1 out]
                    n1010 = stacked-sequence {
                      tunnel: w1333 -> [w1339 _ _]
                      tunnel: w1332 -> [_ w1359 _]
                      tunnel: w1330 -> [w1336 w1356 _]
                      frame #0 {
                        n1011 = global read "Global_Telescopio.vi" "guide_asc"() -> (w1338:dbl)
                        n1012 = local read "AtualDEC"() -> (w1344:dbl)
                        n1013 = global read "Global_Telescopio.vi" "CorrecaoMin"() -> (w1334:dbl)
                        n1014 = Cosine(x=w1344) -> (cos(x)=w1343:dbl)
                        n1015 = Multiply(x=w1338, y=w1336) -> (x*y=w1337:dbl)
                        n1016 = Absolute Value(x=w1343) -> (abs(x)=w1342:dbl)
                        n1017 = Divide(x=w1337, y=w1342) -> (x/y=w1340:dbl)
                        n1018 = Multiply(x=w1339, y=w1340) -> (x*y=w1335:dbl)
                        n1019 = Greater?(x=w1340, y=w1334) -> (0:w1341:bool)
                        n1020 = case shown="True" w1341 {
                          tunnel: w1335 -> [_ w1346]
                          frame False {
                          }
                          frame True {
                            w1350 = u16 1 items=["ZERO", "AH", "DEC", "TUBO", "CUP"] ("Controlador")
                            # "PROCESSO MOVE TELESCÓPIO"
                            n1021 = local read "Offset RA"() -> (w1347:dbl)
                            n1022 = Add(x=w1346, y=w1347) -> (x+y=w1348:dbl)
                            n1023 = property on="Calagem" class="Bool"("Disabled"=u8 2) -> ()  [unwired: 2 in, 2 out]
                            n1024 = call "Conversao Ms to Hora texto.vi"("TRUE=HORA\nFALSE=GRAU"=TRUE ("TRUE=HORA\nFALSE=GRAU"), "PrecDEC"=w1346) -> ("Hora/Graus Texto Decimal"=w1353:string)
                            n1025 = local write "Offset RA"(w1348) -> ()
                            n1026 = call "Monta Comando.vi"("Set Point"=w1353, "Comando"="MOVER_REL", "Dispositivo"="EIXO" ("Comando"), "Controlador"=w1350) -> ()  [unwired: 1 in, 5 out]
                          }
                        }
                      }
                      frame #1 {
                        n1027 = global read "Global_Telescopio.vi" "guide_dec"() -> (w1358:dbl)
                        n1028 = Multiply(x=w1358, y=w1356) -> (x*y=w1357:dbl)
                        n1029 = global read "Global_Telescopio.vi" "CorrecaoMin"() -> (w1354:dbl)
                        n1030 = Greater?(x=w1357, y=w1354) -> (0:w1360:bool)
                        n1031 = Multiply(x=w1359, y=w1357) -> (x*y=w1355:dbl)
                        n1032 = case shown="True" w1360 {
                          tunnel: w1355 -> [_ w1362]
                          frame False {
                          }
                          frame True {
                            w1366 = u16 2 items=["ZERO", "AH", "DEC", "TUBO", "CUP"] ("Controlador")
                            # "PROCESSO MOVE TELESCÓPIO"
                            n1033 = local read "Offset DEC"() -> (w1363:dbl)
                            n1034 = Add(x=w1362, y=w1363) -> (x+y=w1364:dbl)
                            n1035 = property on="Calagem" class="Bool"("Disabled"=u8 2) -> ()  [unwired: 2 in, 2 out]
                            n1036 = call "Conversao Ms to Hora texto.vi"("TRUE=HORA\nFALSE=GRAU"=FALSE ("TRUE=HORA\nFALSE=GRAU"), "PrecDEC"=w1362) -> ("Hora/Graus Texto Decimal"=w1369:string)
                            n1037 = local write "Offset DEC"(w1364) -> ()
                            n1038 = call "Monta Comando.vi"("Set Point"=w1369, "Comando"="MOVER_REL", "Dispositivo"="EIXO" ("Comando"), "Controlador"=w1366) -> ()  [unwired: 1 in, 5 out]
                          }
                        }
                      }
                      frame #2 {
                        # "Reseta Flag da comunicação do Guider"
                        n1039 = global write "Global_Telescopio.vi" "Correção Guider"(FALSE ("Correção Guider")) -> ()
                      }
                    }
                  }
                  frame True {
                    # "20250728"
                    n1040 = global write "Global_Telescopio.vi" "Correção Guider"(FALSE ("Correção Guider")) -> ()
                  }
                }
              }
            }
            n1041 = call "Borda Subida.vi"("Entrada"=w1253) -> ("Boolean"=w1258:bool)  [unwired: 4 in]
            n1042 = Select(t=T5."Disabled and Grayed Out" ("Disabled"), s=w1254, f=T5."Enabled" ("Disabled")) -> (s? t:f=w1256:T5)
            n1043 = property on="ExternalTracking" class="Bool (strict)"("DisabledEnum"=w1256) -> ()  [unwired: 2 in, 2 out]
            n1044 = case shown="True" w1258 {
              frame False {
              }
              frame True {
                n1045 = local write "Offset RA"(0.0 ("Offset RA")) -> ()
                n1046 = local write "Offset DEC"(0.0 ("Offset DEC")) -> ()
              }
            }
            "LED GUIDER" <- "GUIDER"
          }
          frame #11 {
            w1387 = u16 12 items=["Alarme", "Atencao", "Erro", "Ocupado", "Protecao", "Embreagem", "Tracking", "Var. Track", "Rápido", "Ligeiro", "Médio", "Lento", "Em movimento", ""] ("NomeStatus")
            w1386 = u16 12 items=["Alarme", "Atencao", "Erro", "Ocupado", "Protecao", "Embreagem", "Tracking", "Var. Track", "Rápido", "Ligeiro", "Médio", "Lento", "Em movimento", ""] ("NomeStatus")
            # "Aqui era a Global\nLIMITE"
            # "Este teste deve ser executado antes do Frame de enviar\ncomando do sistema de aquisição, em virtude de teste do \nmovimento."
            # "Quando o Movimento Parar\nreseta a Variável/Flag para enviar \no CR ao sitema de Aquisição"
            n1047 = global read "Global_Telescopio.vi" "AQ Offset Mov"() -> (w1383:bool)
            n1048 = call "Bit Status AH.vi"("NomeStatus"=w1386) -> ("StatBit"=w1389:bool)
            n1049 = call "Bit Status DEC.vi"("NomeStatus"=w1387) -> ("StatBit"=w1388:bool)
            n1050 = local read "Proteção"() -> (w1379:bool)
            n1051 = Not Or(1:w1388, 2:w1389) -> (0:w1384:bool)
            n1052 = case shown="True" w1379 {
              selector: w1379 -> [w1390 w1391]
              frame False {
                n1053 = local write "LIMITE"(w1390) -> ()
                n1054 = property on="LIMITE" class="Bool"("Blinking"=w1390) -> ()  [unwired: 2 in, 2 out]
              }
              frame True {
                n1055 = property on="LIMITE" class="Bool"("Blinking"=w1391) -> ()  [unwired: 2 in, 2 out]
                "LIMITE" <- w1391
              }
            }
            n1056 = And(x=w1383, y=w1384) -> (x .and. y?=w1385:bool)
            n1057 = case shown="True" w1385 {
              frame False {
              }
              frame True {
                n1058 = global write "Global_Telescopio.vi" "AQ Offset Mov"(FALSE ("AQ Offset Mov")) -> ()
              }
            }
            n1059 = global read "Global_Telescopio.vi" "Z_SEGURANÇA_GRAUS"() -> (w1382:dbl)
            n1060 = global read "Global_Telescopio.vi" "Zenital angle GRAUS"() -> (w1381:dbl)
            n1061 = global read "Global_Telescopio.vi" "FinalsFileDownload"() -> (→"Precess Data out-of-date":bool)
            n1062 = Greater?(x=w1381, y=w1382) -> (0:→"Security Zone":bool)
          }
          frame #12 {
            w1406 = u16 8 items=["Alarme", "Atencao", "Erro", "Ocupado", "Protecao", "Embreagem", "Tracking", "Var. Track", "Rápido", "Ligeiro", "Médio", "Lento", "Em movimento", ""] ("NomeStatus")
            w1407 = u16 8 items=["Alarme", "Atencao", "Erro", "Ocupado", "Protecao", "Embreagem", "Tracking", "Var. Track", "Rápido", "Ligeiro", "Médio", "Lento", "Em movimento", ""] ("NomeStatus")
            # "TU safe"
            # "ATUALIZAÇÃO DO QUADRO STATUS INFORMATION"
            n1063 = call "Bit Status DEC.vi"("NomeStatus"=w1406) -> ("StatBit"=w1404:bool)
            n1064 = call "Bit Status AH.vi"("NomeStatus"=w1407) -> ("StatBit"=w1405:bool)
            n1065 = Or(x=w1405, y=w1404) -> (x .or. y?=w1403:bool)
            n1066 = case shown="True" w1403 {
              tunnel: [FALSE w1418] -> w1402
              tunnel: [w1408 w1419] -> w1394
              frame False {
                w1412 = u16 10 items=["Alarme", "Atencao", "Erro", "Ocupado", "Protecao", "Embreagem", "Tracking", "Var. Track", "Rápido", "Ligeiro", "Médio", "Lento", "Em movimento", ""] ("NomeStatus")
                w1411 = u16 10 items=["Alarme", "Atencao", "Erro", "Ocupado", "Protecao", "Embreagem", "Tracking", "Var. Track", "Rápido", "Ligeiro", "Médio", "Lento", "Em movimento", ""] ("NomeStatus")
                w1416 = u16 9 items=["Alarme", "Atencao", "Erro", "Ocupado", "Protecao", "Embreagem", "Tracking", "Var. Track", "Rápido", "Ligeiro", "Médio", "Lento", "Em movimento", ""] ("NomeStatus")
                w1417 = u16 9 items=["Alarme", "Atencao", "Erro", "Ocupado", "Protecao", "Embreagem", "Tracking", "Var. Track", "Rápido", "Ligeiro", "Médio", "Lento", "Em movimento", ""] ("NomeStatus")
                n1067 = call "Bit Status AH.vi"("NomeStatus"=w1417) -> ("StatBit"=w1415:bool)
                n1068 = call "Bit Status DEC.vi"("NomeStatus"=w1416) -> ("StatBit"=w1414:bool)
                n1069 = call "Bit Status AH.vi"("NomeStatus"=w1411) -> ("StatBit"=w1410:bool)
                n1070 = call "Bit Status DEC.vi"("NomeStatus"=w1412) -> ("StatBit"=w1409:bool)
                n1071 = Compound Arithmetic op=OR(w1415, w1414, w1410, w1409) -> (w1408:bool)
              }
              frame True {
                w1418 = TRUE
                n1072 = Not(x=w1418) -> (.not. x?=w1419:bool)
              }
            }
            "Mount Gross Movement" <- w1402
            "Mount Fine Movement" <- w1394
            n1073 = global read "Global_Telescopio.vi" "Bit RX Guider"() -> (w1401:bool)
            n1074 = global read "Global_Telescopio.vi" "Bit RX Aquis"() -> (w1400:bool)
            n1075 = case shown="True" w1401 {
              selector: w1401 -> [w1431 w1432]
              frame False {
                n1076 = local write "Auto guider Activity"(w1431) -> ()
              }
              frame True {
                # "Liga Led RX por 1 ciclo"
                n1077 = global write "Global_Telescopio.vi" "Bit RX Guider"(FALSE) -> ()
                "Auto guider Activity" <- w1432
              }
            }
            n1078 = case shown="True" w1400 {
              selector: w1400 -> [w1428 w1430]
              frame False {
                n1079 = local write "Data Acquisition Activity"(w1428) -> ()
              }
              frame True {
                # "Liga Led RX por 1 ciclo"
                n1080 = global write "Global_Telescopio.vi" "Bit RX Aquis"(FALSE) -> ()
                "Data Acquisition Activity" <- w1430
              }
            }
            n1081 = case shown="True" "News" {
              selector: "News" -> [_ w1424]
              frame False {
              }
              frame True {
                n1082 = flat-sequence {
                  tunnel: w1424 -> [w1425]
                  frame #0 {
                    n1083 = call "Monta_Mensagem.vi"("Zerar"=w1425) -> ()  [unwired: 2 in]
                  }
                  frame #1 {
                    n1084 = global write "Global_Telescopio.vi" "SYSTEM MESSAGES"("Removida dependência NI VISION. Build com LabVIEW 2018.\nComunicação com a estação meteorológica passou a ter parâmetros configuráveis, sinalização do recebimento dos dados e recuperação automática da conexão. Verificação do formato das coordenadas de apontamento digitadas pelo usuário. Corrigido bug de travamento de DEC no final de um apontamento. " ("SYSTEM MESSAGES")) -> ()
                  }
                }
              }
            }
            n1085 = global read "Global_Telescopio.vi" "SYSTEM MESSAGES"() -> (→"SYSTEM MESSAGES":string)
            n1086 = case shown="True" "Clear All Messages" {
              selector: "Clear All Messages" -> [_ w1427]
              frame False {
              }
              frame True {
                n1087 = call "Monta_Mensagem.vi"("Zerar"=w1427) -> ()  [unwired: 2 in]
                n1088 = call "Monta_Mensagem.vi"("Zerar"=w1427) -> ()  [unwired: 2 in]
              }
            }
            n1089 = local read "alarm Time"() -> (w1395:timestamp)
            n1090 = call "Get host time.vi"() -> ("BR current time"=w1393:timestamp)  [unwired: 8 in, 3 out]
            n1091 = Greater?(x=w1393, y=w1395) -> (0:w1396:bool)
            n1092 = case shown="True" w1396 {
              frame False {
              }
              frame True {
                n1093 = local read "Flag Alarm"() -> (w1420:bool)
